vi "[FPGA] SAR Acq Main.vi"() -> ()   [LabVIEW 2017]
doc: "This VI provides a template for customizing a waveform acquisition using scanned (or SAR) based NI C Series analog input modules."
uses:
  <vilib>/Platform/TimedLoop/XDataNode/timing_clust.ctl
  <vilib>/Platform/TimedLoop/XDataNode/nitl_modes.ctl
  <vilib>/Platform/TimedLoop/XDataNode/wakeup.ctl
  <instrlib>/_niInstr/Instruction Framework/v1/FPGA/Helper Classes/Single Address Space Collection/Single Address Space Collection.lvclass
  C:/Program Files (x86)/National Instruments/LabVIEW 2017/instr.lib/_niInstr/Instruction Framework/v1/FPGA/Interfaces/Address Space Collection/Address Space Collection.lvclass
  <instrlib>/_niInstr/FIFO Register Bus/v1/FPGA/niInstr FIFO Register Bus v1 FPGA.lvclass
  C:/Program Files (x86)/National Instruments/LabVIEW 2017/instr.lib/_niInstr/Instruction Framework/v1/FPGA/Interfaces/Instruction Producer/Instruction Producer.lvclass
  <vilib>/rvi/Emulation/niFpgaGetClockAttributes.vi
  <vilib>/rvi/Emulation/niFpgaSctlEmulationGetInTimedLoop.vi
  <vilib>/rvi/Emulation/niFpgaEmulationReportErrorSimple.vi
  <vilib>/rvi/Emulation/niFpgaCriticalErrorInLSC.vi
  <vilib>/Platform/TimedLoop/XDataNode/XDataNode.xnode
  WaveformAddressSpace.lvclass
  <vilib>/Platform/TimedLoop/XDataNode/XDNodeRunTimeDep.lvlib
  <instrlib>/_niInstr/Instruction Framework/v1/FPGA/Top Level Bus/Register Configuration/Register Configuration.lvclass
panel:
  in  "injectError0":errorcluster
  in  "fifo reg bus ctrl 0":u32
  out "fifo reg bus status 0":u32
  out "fifo reg bus data 0":u64
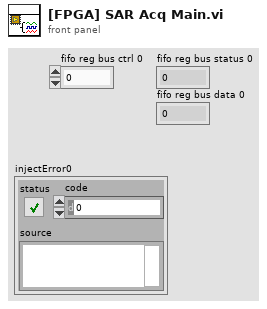
[diagram p1: front panel]
types:
  T1 = typedef "XDNodeRunTimeDep.lvlib/timing_clust.ctl" = cluster{"Expected End [f-1]":u64, "Actual End [f-1]":u64, "Finished Late? [f-1]":bool, "Expected End [i-1]":u64, "Actual End [i-1]":u64, "Finished Late? [i-1]":bool, "Expected Start [i]":u64, "Actual Start [i]":u64, "Expected Start [f]":u64, "Actual Start [f]":u64, "Source Name":string, "Structure Name":string, "Period":i64, "Deadline":i64, "Offset":i64, "Start":i64, "Priority":i32, "Timeout":i32, "Mode":T2, "Wakeup Reason":T3, "Error":errorcluster, "Source Type":string, "Secondary Source Type":string, "Global End Time":u64, "Global Start Time":u64, "Frame Duration":u64, "Iteration Duration":u64, "Assigned CPU":i32, "I/O Scan Engine Mode":u32}
  T2 = typedef "XDNodeRunTimeDep.lvlib/nitl_modes.ctl" = enum32{"No Change", "Process missed periods, maintain original phase", "Discard missed periods, maintain original phase", "Process missed periods, ignore original phase", "Discard missed periods, ignore original phase"}
  T3 = typedef "XDNodeRunTimeDep.lvlib/wakeup.ctl" = enum32{"Normal", "Aborted", "Asynchronous wakeup", "Timing source error", "Timed loop error", "Timeout"}
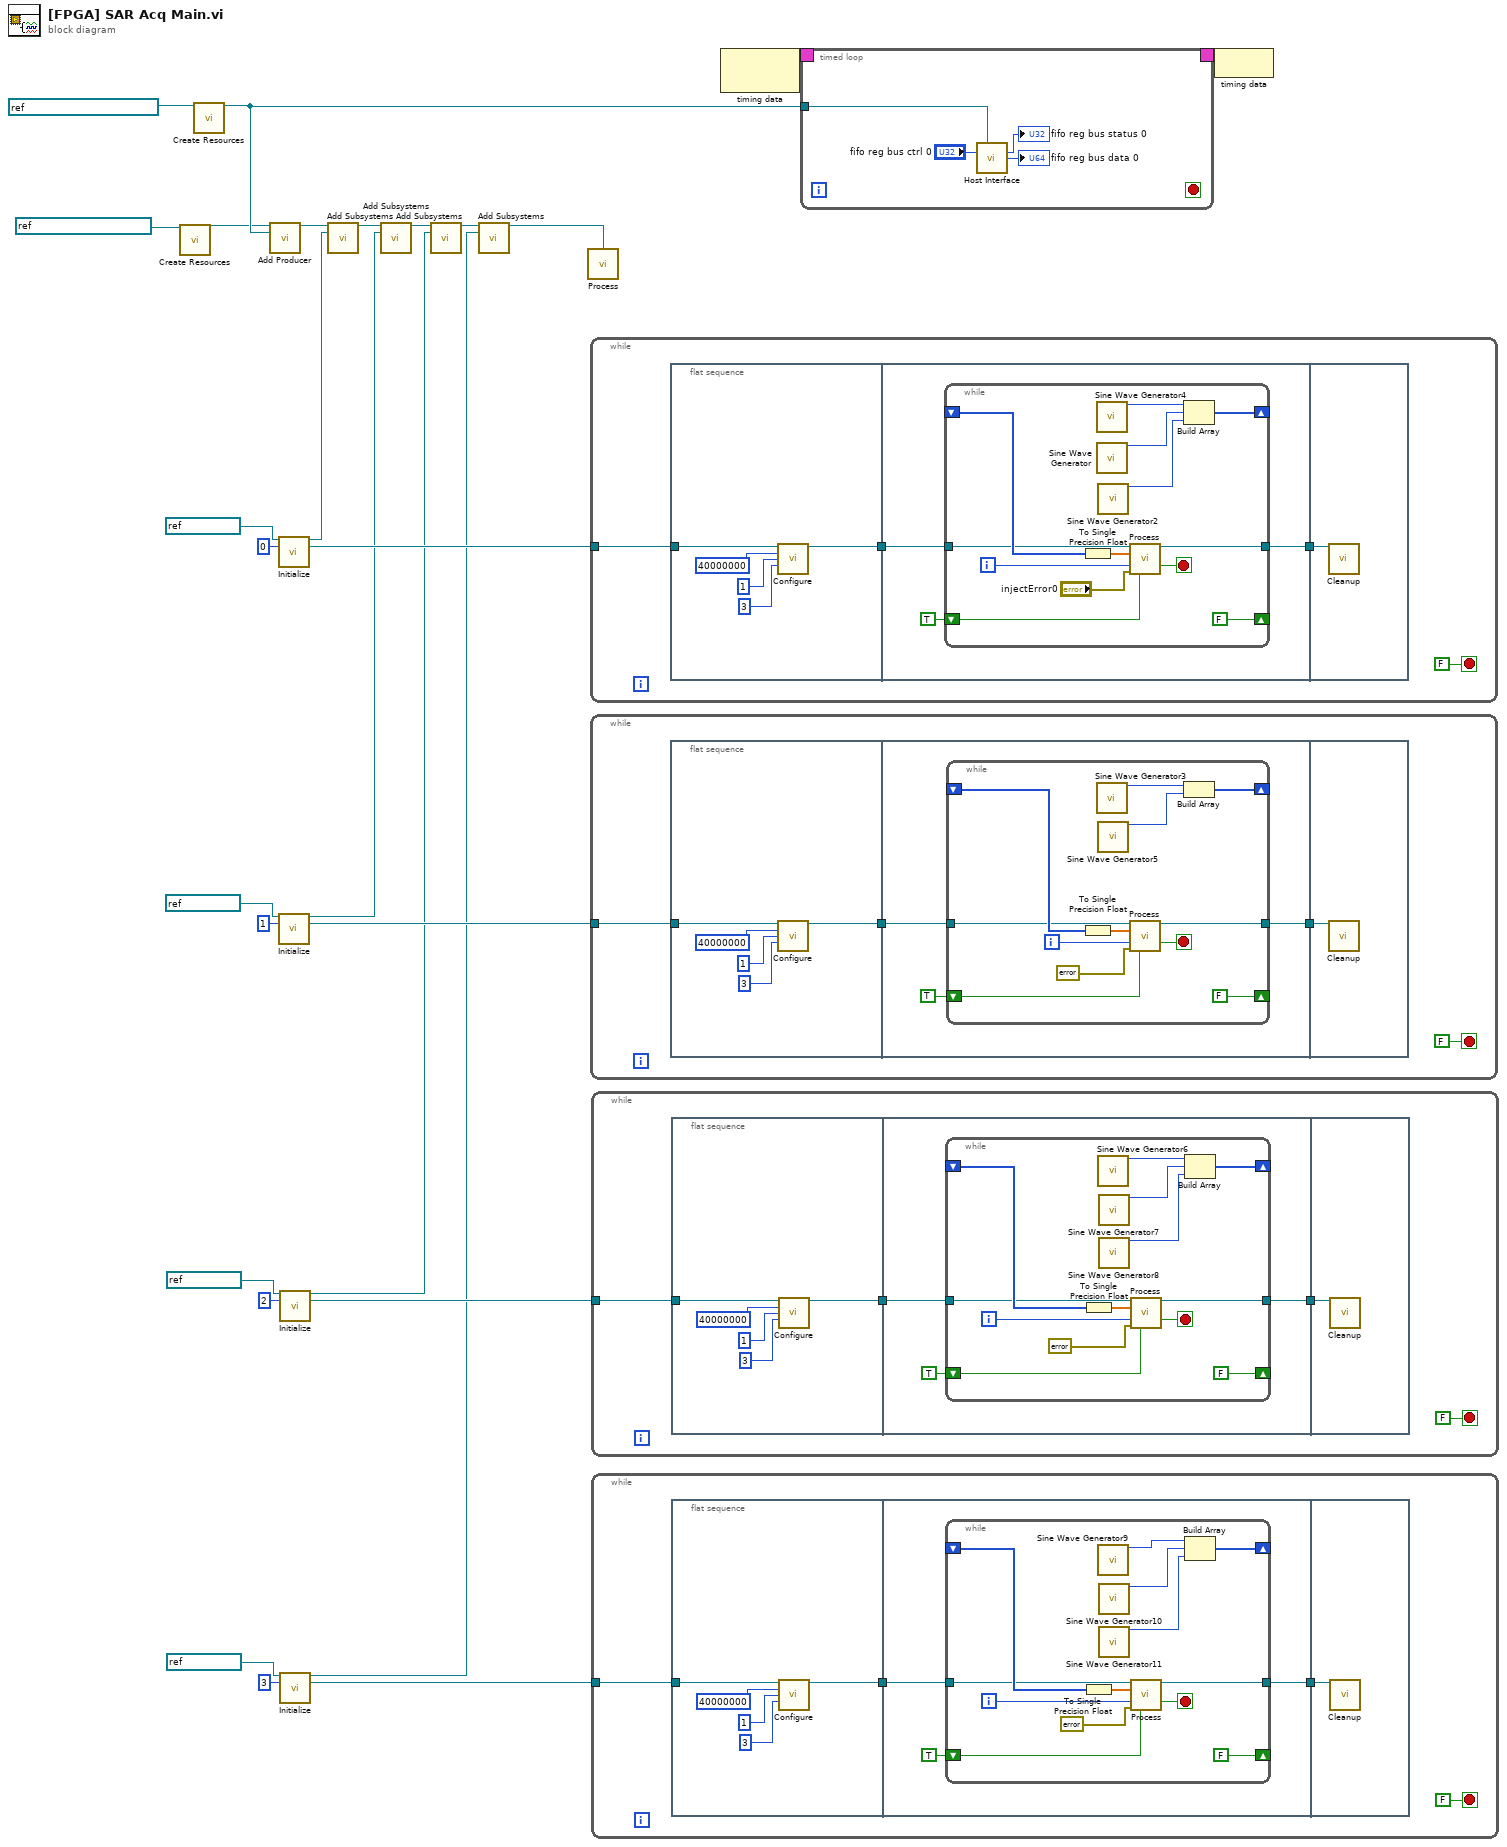
[diagram p0: block diagram]
diagram:
  n1 = call <instrlib>:"Create Resources.vi"("register clock"=refnum<k21> "40 MHz Onboard Clock") -> ("register configuration"=w23:refnum<class "Register Configuration.lvclass">)  [unwired: 14 in]
  n2 = call <instrlib>:"Create Resources.vi"("instruction fifo"=refnum<k21> "reg.host instruction fifo 0") -> ("fifo register bus"=w24:refnum<class "niInstr FIFO Register Bus v1 FPGA.lvclass">)  [unwired: 14 in]
  n3 = call <instrlib>:"Add Producer.vi"("register configuration in"=w23, "instruction producer"=w24) -> ("register configuration out"=w21:refnum<class "Register Configuration.lvclass">)  [unwired: 13 in]
  n4 = call "Initialize.vi"("DMA FIFO"=refnum<k21> "DataSGL0" ("FIFO Out"), "instance"=u8 0) -> ("subsystem"=w14:refnum<class "Single Address Space Collection.lvclass">, "AddressSpace"=w15:refnum<class "WaveformAddressSpace.lvclass">)  [unwired: 12 in]
  n5 = call "Initialize.vi"("DMA FIFO"=refnum<k21> "DataSGL1" ("FIFO Out"), "instance"=u8 1) -> ("subsystem"=w9:refnum<class "Single Address Space Collection.lvclass">, "AddressSpace"=w12:refnum<class "WaveformAddressSpace.lvclass">)  [unwired: 12 in]
  n6 = call "Initialize.vi"("DMA FIFO"=refnum<k21> "DataSGL2" ("FIFO Out"), "instance"=u8 2) -> ("subsystem"=w5:refnum<class "Single Address Space Collection.lvclass">, "AddressSpace"=w6:refnum<class "WaveformAddressSpace.lvclass">)  [unwired: 12 in]
  n7 = call "Initialize.vi"("DMA FIFO"=refnum<k21> "DataSGL3" ("FIFO Out"), "instance"=u8 3) -> ("subsystem"=w1:refnum<class "Single Address Space Collection.lvclass">, "AddressSpace"=w4:refnum<class "WaveformAddressSpace.lvclass">)  [unwired: 12 in]
  n8 = call <instrlib>:"Add Subsystems.vi"("register configuration in"=w21, "subsystems"=w14) -> ("register configuration out"=w20:refnum<class "Register Configuration.lvclass">)  [unwired: 13 in]
  n9 = call <instrlib>:"Add Subsystems.vi"("register configuration in"=w20, "subsystems"=w9) -> ("register configuration out"=w19:refnum<class "Register Configuration.lvclass">)  [unwired: 13 in]
  n10 = call <instrlib>:"Add Subsystems.vi"("register configuration in"=w19, "subsystems"=w5) -> ("register configuration out"=w18:refnum<class "Register Configuration.lvclass">)  [unwired: 13 in]
  n11 = call <instrlib>:"Add Subsystems.vi"("register configuration in"=w18, "subsystems"=w1) -> ("register configuration out"=w13:refnum<class "Register Configuration.lvclass">)  [unwired: 13 in]
  n12 = call <instrlib>:"Process.vi"("register configuration"=w13) -> ()  [unwired: 15 in]
  n13 = while {
    tunnel: w15 -> [w28]
    stop <- FALSE stop-if-true
    n14 = flat-sequence {
      tunnel: [w32] -> w30
      tunnel: w28 -> [w33]
      tunnel: w30 -> [w39]
      tunnel: [w38] -> w29
      tunnel: w29 -> [w53]
      frame #0 {
        n15 = call "Configure.vi"("WaveformAddressSpace in"=w33, "oclk_freq"=u32 40000000, "oclk_mult"=u32 1, "UnderflowMargin"=u32 3 ("y")) -> ("WaveformAddressSpace out"=w32:refnum<class "WaveformAddressSpace.lvclass">)  [unwired: 11 in]
      }
      frame #1 {
        n16 = while {
          shift-right: [w49] -> _
          shift-left: _ -> [w51]
          shift-right: [FALSE] -> _
          shift-left: TRUE -> [w40]
          tunnel: w39 -> [w44]
          tunnel: [w43] -> w38
          i -> [w50]
          stop <- w46 stop-if-true
          n17 = To Single Precision Float(number=w51) -> (single precision float=w45:sgl[])
          n18 = call "Sine Wave Generator4"() -> ("sine out"=w48:i16)  [unwired: 15 in]
          n19 = call "Sine Wave Generator"() -> ("sine out"=w42:i16)  [unwired: 15 in]
          n20 = call "Sine Wave Generator2"() -> ("sine out"=w41:i16)  [unwired: 15 in]
          n21 = call <instrlib>:"Process.vi"("WaveformAddressSpace in"=w44, "Data"=w45, "Iteration"=w50, "error in (no error)"="injectError0", "FirstIteration"=w40) -> ("WaveformAddressSpace out"=w43:refnum<class "WaveformAddressSpace.lvclass">, "stop"=w46:bool)  [unwired: 7 in, 2 out]
          n22 = Build Array(w48, w42, w41) -> (w49:i16[])
        }
      }
      frame #2 {
        n23 = call "Cleanup.vi"("WaveformAddressSpace in"=w53) -> ()  [unwired: 14 in, 1 out]
      }
    }
  }
  n24 = while {
    tunnel: w12 -> [w54]
    stop <- FALSE stop-if-true
    n25 = flat-sequence {
      tunnel: [w58] -> w56
      tunnel: w54 -> [w59]
      tunnel: w56 -> [w65]
      tunnel: [w64] -> w55
      tunnel: w55 -> [w78]
      frame #0 {
        n26 = call "Configure.vi"("WaveformAddressSpace in"=w59, "oclk_freq"=u32 40000000, "oclk_mult"=u32 1, "UnderflowMargin"=u32 3 ("y")) -> ("WaveformAddressSpace out"=w58:refnum<class "WaveformAddressSpace.lvclass">)  [unwired: 11 in]
      }
      frame #1 {
        n27 = while {
          shift-right: [w74] -> _
          shift-left: _ -> [w76]
          shift-right: [FALSE] -> _
          shift-left: TRUE -> [w66]
          tunnel: w65 -> [w69]
          tunnel: [w68] -> w64
          i -> [w75]
          stop <- w71 stop-if-true
          n28 = To Single Precision Float(number=w76) -> (single precision float=w70:sgl[])
          n29 = call "Sine Wave Generator3"() -> ("sine out"=w73:i16)  [unwired: 15 in]
          n30 = call "Sine Wave Generator5"() -> ("sine out"=w67:i16)  [unwired: 15 in]
          n31 = call <instrlib>:"Process.vi"("WaveformAddressSpace in"=w69, "Data"=w70, "Iteration"=w75, "error in (no error)"=errorcluster {"status"=FALSE, "code"=0, "source"=""} ("injectError1"), "FirstIteration"=w66) -> ("WaveformAddressSpace out"=w68:refnum<class "WaveformAddressSpace.lvclass">, "stop"=w71:bool)  [unwired: 7 in, 2 out]
          n32 = Build Array(w73, w67) -> (w74:i16[])
        }
      }
      frame #2 {
        n33 = call "Cleanup.vi"("WaveformAddressSpace in"=w78) -> ()  [unwired: 14 in, 1 out]
      }
    }
  }
  n34 = while {
    tunnel: w6 -> [w79]
    stop <- FALSE stop-if-true
    n35 = flat-sequence {
      tunnel: [w83] -> w81
      tunnel: w79 -> [w84]
      tunnel: w81 -> [w90]
      tunnel: [w89] -> w80
      tunnel: w80 -> [w104]
      frame #0 {
        n36 = call "Configure.vi"("WaveformAddressSpace in"=w84, "oclk_freq"=u32 40000000, "oclk_mult"=u32 1, "UnderflowMargin"=u32 3 ("y")) -> ("WaveformAddressSpace out"=w83:refnum<class "WaveformAddressSpace.lvclass">)  [unwired: 11 in]
      }
      frame #1 {
        n37 = while {
          shift-right: [w100] -> _
          shift-left: _ -> [w102]
          shift-right: [FALSE] -> _
          shift-left: TRUE -> [w91]
          tunnel: w90 -> [w95]
          tunnel: [w94] -> w89
          i -> [w101]
          stop <- w97 stop-if-true
          n38 = To Single Precision Float(number=w102) -> (single precision float=w96:sgl[])
          n39 = call "Sine Wave Generator6"() -> ("sine out"=w99:i16)  [unwired: 15 in]
          n40 = call "Sine Wave Generator7"() -> ("sine out"=w93:i16)  [unwired: 15 in]
          n41 = call "Sine Wave Generator8"() -> ("sine out"=w92:i16)  [unwired: 15 in]
          n42 = call <instrlib>:"Process.vi"("WaveformAddressSpace in"=w95, "Data"=w96, "Iteration"=w101, "error in (no error)"=errorcluster {"status"=FALSE, "code"=0, "source"=""} ("injectError2"), "FirstIteration"=w91) -> ("WaveformAddressSpace out"=w94:refnum<class "WaveformAddressSpace.lvclass">, "stop"=w97:bool)  [unwired: 7 in, 2 out]
          n43 = Build Array(w99, w93, w92) -> (w100:i16[])
        }
      }
      frame #2 {
        n44 = call "Cleanup.vi"("WaveformAddressSpace in"=w104) -> ()  [unwired: 14 in, 1 out]
      }
    }
  }
  n45 = while {
    tunnel: w4 -> [w105]
    stop <- FALSE stop-if-true
    n46 = flat-sequence {
      tunnel: [w109] -> w107
      tunnel: w105 -> [w110]
      tunnel: w107 -> [w116]
      tunnel: [w115] -> w106
      tunnel: w106 -> [w130]
      frame #0 {
        n47 = call "Configure.vi"("WaveformAddressSpace in"=w110, "oclk_freq"=u32 40000000, "oclk_mult"=u32 1, "UnderflowMargin"=u32 3 ("y")) -> ("WaveformAddressSpace out"=w109:refnum<class "WaveformAddressSpace.lvclass">)  [unwired: 11 in]
      }
      frame #1 {
        n48 = while {
          shift-right: [w126] -> _
          shift-left: _ -> [w128]
          shift-right: [FALSE] -> _
          shift-left: TRUE -> [w117]
          tunnel: w116 -> [w121]
          tunnel: [w120] -> w115
          i -> [w127]
          stop <- w123 stop-if-true
          n49 = To Single Precision Float(number=w128) -> (single precision float=w122:sgl[])
          n50 = call "Sine Wave Generator9"() -> ("sine out"=w125:i16)  [unwired: 15 in]
          n51 = call "Sine Wave Generator10"() -> ("sine out"=w119:i16)  [unwired: 15 in]
          n52 = call "Sine Wave Generator11"() -> ("sine out"=w118:i16)  [unwired: 15 in]
          n53 = call <instrlib>:"Process.vi"("WaveformAddressSpace in"=w121, "Data"=w122, "Iteration"=w127, "error in (no error)"=errorcluster {"status"=FALSE, "code"=0, "source"=""} ("injectError3"), "FirstIteration"=w117) -> ("WaveformAddressSpace out"=w120:refnum<class "WaveformAddressSpace.lvclass">, "stop"=w123:bool)  [unwired: 7 in, 2 out]
          n54 = Build Array(w125, w119, w118) -> (w126:i16[])
        }
      }
      frame #2 {
        n55 = call "Cleanup.vi"("WaveformAddressSpace in"=w130) -> ()  [unwired: 14 in, 1 out]
      }
    }
  }
  n56 = node-c288() -> (w27:T1)  [unwired: 1 in]
  n57 = timed-loop {
    timing: w27 -> [_]
    timing-out: [_] -> w26
    tunnel: w24 -> [w134]
    stop <- _ stop-if-true
    n58 = call <instrlib>:"Host Interface.vi"("fifo register bus"=w134, "fifo reg bus ctrl 0"="fifo reg bus ctrl 0") -> ("fifo reg bus status 0"=→"fifo reg bus status 0":u32, "fifo reg bus data 0"=→"fifo reg bus data 0":u64)  [unwired: 12 in]
  }
  n59 = node-c288(w26) -> ()
